vi "ResetQueue.vi"(8 "error constant":errorcluster) -> (0 "error constant 2":errorcluster)   [LabVIEW 2019]
uses:
  GraphsQueue.vi
  Global.lvlib
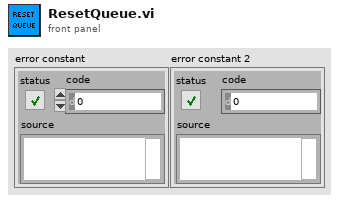
[diagram p1: front panel]
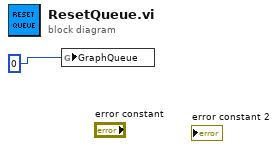
[diagram p0: block diagram]
diagram:
  n1 = global write "GraphsQueue.vi" "GraphQueue"(i16 0 ("GraphQueue")) -> ()
